vi "Joystick Deadband.vi"(1 "Stick In":dbl) -> (0 "Stick Out":dbl)   [LabVIEW 2014]
uses:
  Robot Code/Robot Global Data.vi
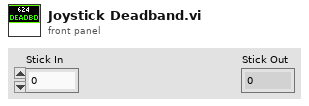
[diagram p1: front panel]
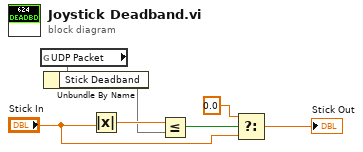
[diagram p0: block diagram]
diagram:
  n1 = global read "Robot Global Data.vi" "UDP Packet"() -> (w1)
  n2 = Unbundle By Name(w1) -> ("Stick Deadband"=w2)
  n3 = Absolute Value(x="Stick In") -> (abs(x)=w7:dbl)
  n4 = Less Or Equal?(x=w7, y=w2) -> (x <= y?=w6:bool)
  n5 = Select(t=0.0, s=w6, f="Stick In") -> (s? t:f=→"Stick Out":dbl)
